vi "Write Application Errors.vi"(8 "error in (no error)":errorcluster, 10 "Application Errors":path, 11 "Error in":refnum<class "Error.lvclass">) -> (0 "error out":errorcluster, 3 "Error out":refnum<class "Error.lvclass">)   [LabVIEW 2019, in "TSC Error.lvlib" / "Error.lvclass"]
doc: "Data Member Access to write the location for the custom errors of the application.\n\nInputs:\n-Error in [obj] - the dynamic dispatch input class\n-Application Errors [path] - the data member access input\n-error in\n\nOutputs:\n-Error out [obj] - the dynamic dispatch output class\n-error out\n________________________________________________________________________________\n<b>Code Developed By:</b>\nDaniel Coons\nTechnology Service Corporation\n1983 S Liberty Drive\nBloomington, IN 47403\nPhone: 812 558-7100\ndaniel.coons@tsc.com\nwww.tsc.com\n\n<b>Date Created:</b> 04 APR 2016\n<b>Date Updated:</b>"
uses:
  Error.lvclass
  Error.lvclass/Error.ctl
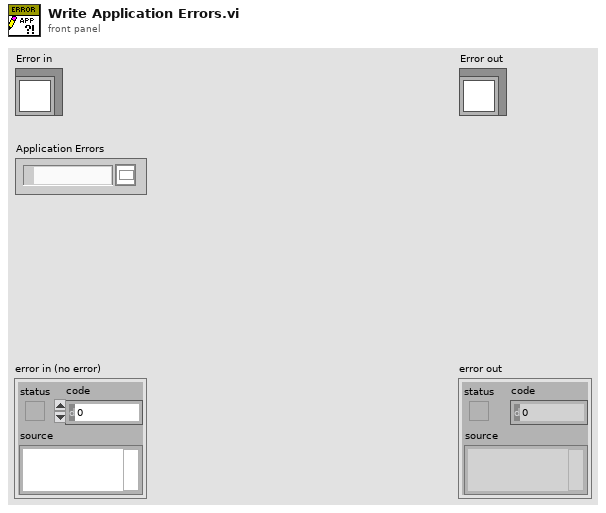
[diagram p1: front panel]
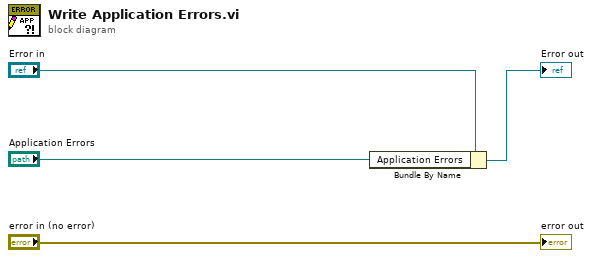
[diagram p0: block diagram]
diagram:
  n1 = Bundle By Name(cluster="Error in", "Application Errors"="Application Errors") -> (→"Error out":refnum<class "Error.lvclass">)
  "error out" <- "error in (no error)"
